vi "Autosort Remove Sort Option.vi"(8 "error in (no error)":errorcluster, 11 "Index":i32) -> (0 "error out":errorcluster)   [LabVIEW 2016]
uses:
  Autosort Parameters Set.vi
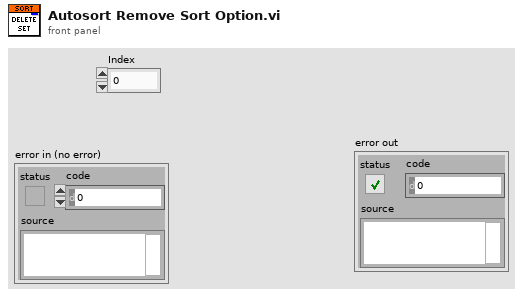
[diagram p1: front panel]
types:
  T1 = enum16{"open", "replace", "create", "open or create", "replace or create", "replace or create with confirmation"}
  T2 = typedef "Autosort Parameters.ctl" = cluster{"Name":string, "Min Vel":dbl, "Trigger Ch":i32, "MaxVel":dbl, "Width":i32, "Pre Impuls":i32, "Post Impuls":i32, "Pitch":dbl, "Other Trigger":bool, "Cross Corr":bool}
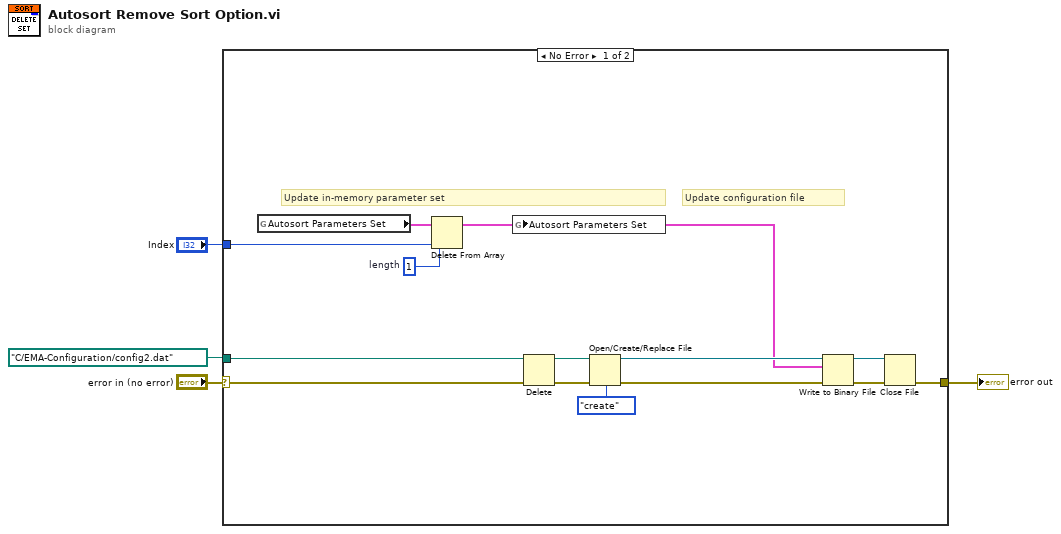
[diagram p0: block diagram]
diagram:
  n1 = case shown="No Error" "error in (no error)" {
    selector: "error in (no error)" -> [w9 w19]
    tunnel: [w6 w19] -> w3
    tunnel: "Index" -> [w17 _]
    tunnel: path "C:/EMA-Configuration/config2.dat" ("path") -> [w10 _]
    frame No Error {
      w16 = 1  # length
      # "Update configuration file"
      # "Update in-memory parameter set"
      n2 = global read "Autosort Parameters Set.vi" "Autosort Parameters Set"() -> (w18:T2[])
      n3 = Delete From Array(array=w18, length=w16, index=w17) -> (array with subset deleted=w8:T2[])  [unwired: 1 out]
      n4 = global write "Autosort Parameters Set.vi" "Autosort Parameters Set"(w8) -> ()
      n5 = Delete(path (use dialog)=w10, error in=w9) -> (deleted path=w15:path, error out=w14:errorcluster)  [unwired: 3 in, 1 out]
      n6 = Open/Create/Replace File(file path (use dialog)=w15, error in=w14, operation (0:open)=T1."create") -> (refnum out=w12:refnum<file>, error out=w11:errorcluster)  [unwired: 3 in, 1 out]
      n7 = Write to Binary File(file (use dialog)=w12, data=w8, error in=w11) -> (refnum out=w5:refnum<file>, error out=w7:errorcluster)  [unwired: 3 in, 1 out]
      n8 = Close File(refnum=w5, error in=w7) -> (error out=w6:errorcluster)  [unwired: 1 out]
    }
    frame Error {
    }
  }
  "error out" <- w3
